vi "Set Error.vi"(4 "Message Postfix":string, 5 "Error Messages":string[](array[string]), 6 "Error Code":i32, 7 "Error Name":string, 8 "error in (no error)":errorcluster, 9 "Ignore CallChain":u16, 11 "Actor in":refnum<class "Ancestral Actor.lvclass">) -> (0 "error out":errorcluster, 3 "Actor out":refnum<class "Ancestral Actor.lvclass">)   [LabVIEW 2016, in "Stream Actor.lvlib" / "Ancestral Actor.lvclass"]
doc: "--\nCopyright © 2017 Composed SystemsI All rights reserved.\n\nAuthor: Jon McBee <jon.mcbee@composed.io>\n\nThis library is provided \"AS IS\" ,WITHOUT WARRANTIES OR\nCONDITIONS OF ANY KIND, either express or implied.\n\nComposed Systems -- composed.io\n\nStream 0.0.1.1\nJon McBee - Composed Systems\nCopyright (c) 2017, Composed Systems"
uses:
  <userlib>/Composed Systems/Stream/Actor/Actor Class/Ancestral Actor.lvclass
  <userlib>/Composed Systems/Stream/Actor/Actor Class/Ancestral Actor.lvclass/Ancestral Actor.ctl
  <userlib>/Composed Systems/Stream/Error/Classes/Error Interface/Error Interface.lvclass
  <userlib>/Composed Systems/Stream/Error/Classes/Application Error/Application Error.lvclass
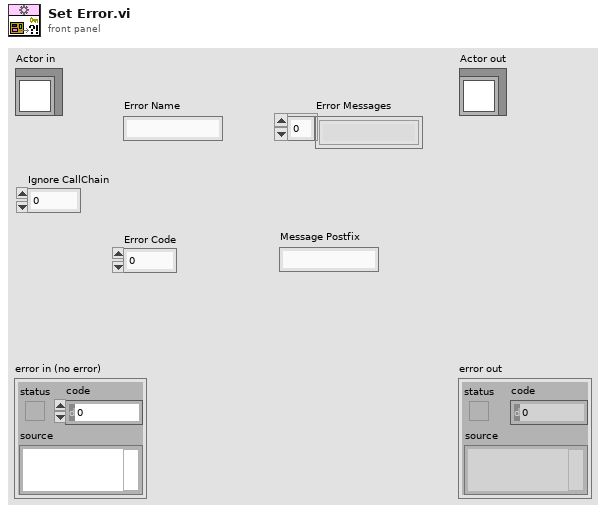
[diagram p1: front panel]
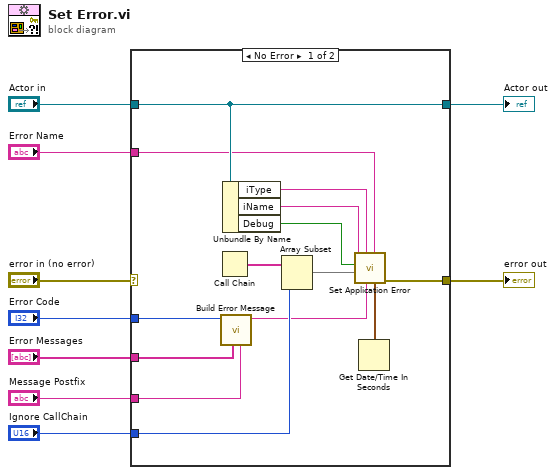
[diagram p0: block diagram]
diagram:
  n1 = case shown="No Error" "error in (no error)" {
    selector: "error in (no error)" -> [_ w25]
    tunnel: [w15 w25] -> w8
    tunnel: [w23 w24] -> w6
    tunnel: "Actor in" -> [w23 w24]
    tunnel: "Error Name" -> [w10 _]
    tunnel: "Error Code" -> [w20 _]
    tunnel: "Error Messages" -> [w19 _]
    tunnel: "Message Postfix" -> [w18 _]
    tunnel: "Ignore CallChain" -> [w21 _]
    frame No Error {
      n2 = Call Chain() -> (call chain=w22:string[])
      n3 = call <userlib>:"Build Error Message.vi"("Message Postfix"=w18, "Error Messages"=w19, "Error Code"=w20) -> ("Error Message"=w17:string)  [unwired: 8 in]
      n4 = Unbundle By Name(w23) -> ("iType"=w11:string, "iName"=w12:string, "Debug"=w13:bool)
      n5 = Array Subset(array=w22, index=w21) -> (w14:string[])  [unwired: 1 in]
      n6 = Get Date/Time In Seconds() -> (seconds since 1Jan1904=w16:timestamp)
      n7 = call <userlib>:"Set Application Error.vi"("Time Stamp"=w16, "Error Name"=w10, "Error Message"=w17, "Error Scope"=w11, "Call Chain"=w14, "Log Error?"=w13, "Error Source"=w12) -> ("Error Out"=w15:errorcluster)  [unwired: 4 in]
    }
    frame Error {
    }
  }
  "error out" <- w8
  "Actor out" <- w6
